vi "Add Resource.vi"   [LabVIEW 2015, in "niInstr AXI4-Stream Writer v1 FPGA.lvclass"]
doc: "Adds a resource to the AXI4-Stream Writer.\n\n<b>Do not place this VI into a case structure or it will not compile correctly!</b>"
uses:
  <instrlib>/_niInstr/CLIP Adapters/v1/FPGA/AXI4-Stream/Writer/niInstr AXI4-Stream Writer v1 FPGA.lvclass
  <instrlib>/_niInstr/CLIP Adapters/v1/FPGA/AXI4-Stream/Writer FXP64x4/niInstr AXI4-Stream Writer FXP64x4 v1 FPGA.lvclass
  <instrlib>/_niInstr/CLIP Adapters/v1/FPGA/AXI4-Stream/Writer FXP64x2/niInstr AXI4-Stream Writer FXP64x2 v1 FPGA.lvclass
  <instrlib>/_niInstr/CLIP Adapters/v1/FPGA/AXI4-Stream/Writer FXP64x1/niInstr AXI4-Stream Writer FXP64x1 v1 FPGA.lvclass
  <instrlib>/_niInstr/CLIP Adapters/v1/FPGA/AXI4-Stream/Writer FXP32x1/niInstr AXI4-Stream Writer FXP32x1 v1 FPGA.lvclass
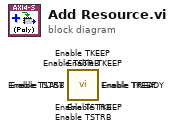
[diagram p0: block diagram]
diagram:
  n1 = call <instrlib>:"Enable TSTRB.vi"() -> ()  [unwired: 11 in, 1 out]
  n2 = call <instrlib>:"Enable TKEEP.vi"() -> ()  [unwired: 11 in, 1 out]
  n3 = call <instrlib>:"Enable TSTRB.vi"() -> ()  [unwired: 11 in, 1 out]
  n4 = call <instrlib>:"Enable TKEEP.vi"() -> ()  [unwired: 11 in, 1 out]
  n5 = call <instrlib>:"Enable TSTRB.vi"() -> ()  [unwired: 11 in, 1 out]
  n6 = call <instrlib>:"Enable TKEEP.vi"() -> ()  [unwired: 11 in, 1 out]
  n7 = call <instrlib>:"Enable TSTRB.vi"() -> ()  [unwired: 11 in, 1 out]
  n8 = call <instrlib>:"Enable TKEEP.vi"() -> ()  [unwired: 11 in, 1 out]
  n9 = call <instrlib>:"Enable TREADY.vi"() -> ()  [unwired: 11 in, 1 out]
  n10 = call <instrlib>:"Enable TLAST.vi"() -> ()  [unwired: 11 in, 1 out]
